vi "CRYReport Part ObjectClicked Event Callback.vi"(4 "TXTextControl":refnum<k7>, 5 "Event Data":cluster{"ObjectId":i16}, 6 "Control Ref":refnum<k7>, 7 "Event Common Data":T1) -> ()   [LabVIEW 2013]
uses:
  CRYReport Global.vi
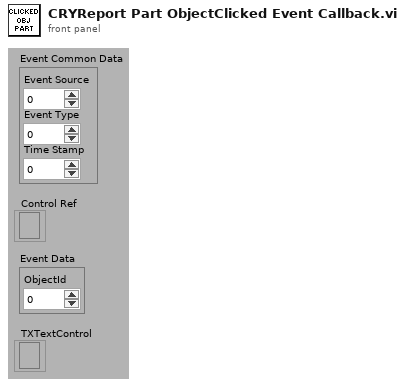
[diagram p1: front panel]
types:
  T1 = cluster{"Event Source":i32, "Event Type":u32, "Time Stamp":u32}
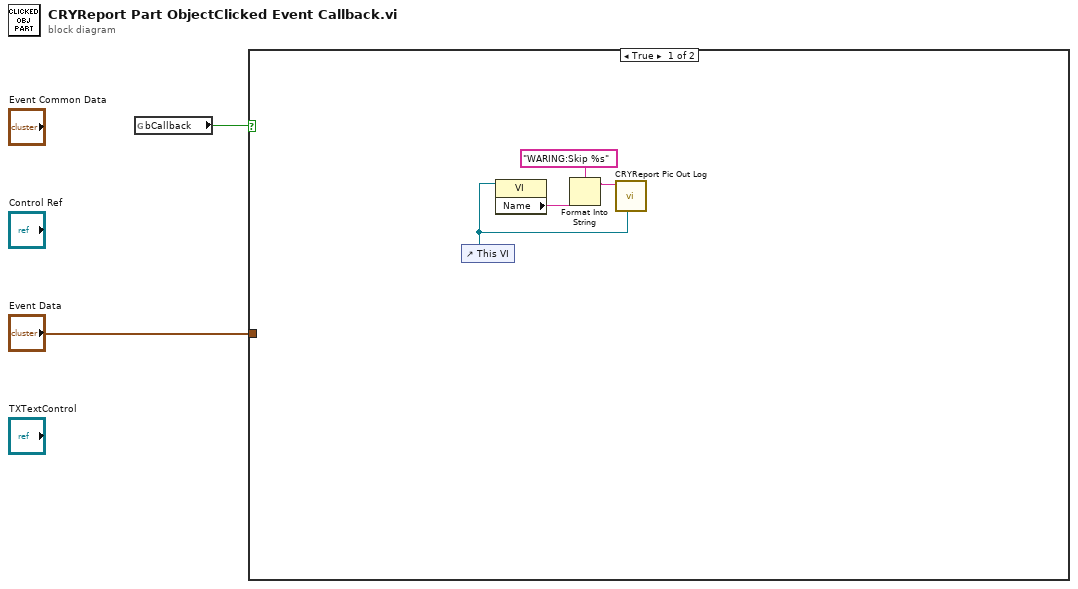
[diagram p0: block diagram]
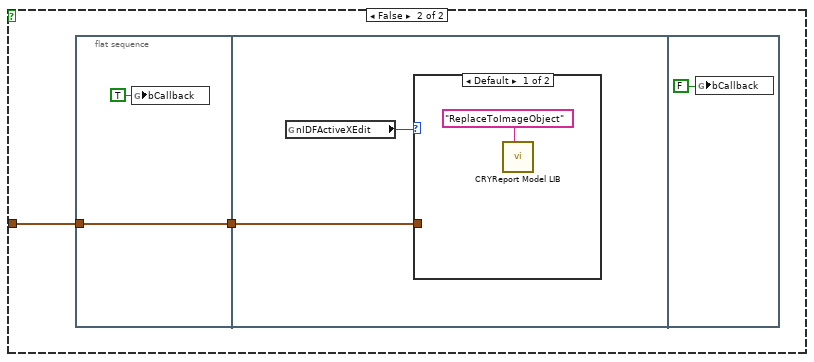
[diagram p2: hidden frame]
diagram:
  n1 = global read "CRYReport Global.vi" "bCallback"() -> (w1:bool)
  n2 = case shown="True" w1 {
    tunnel: "Event Data" -> [_ w7]
    frame True {
      n3 = control-ref of="This VI"() -> (w3:refnum<vi>)
      n4 = property class="VI"(reference=w3) -> ("Name"=w4:string)  [unwired: 1 in, 2 out]
      n5 = Format Into String(format string="WARING:Skip %s" ("string"), w4) -> (resulting string=w6:string)  [unwired: 2 in, 1 out]
      n6 = call "CRYReport Pic Out Log.vi"("vi reference"=w3, "sData"=w6) -> ()  [unwired: 10 in]
    }
    frame False {
      n7 = flat-sequence {
        tunnel: w7 -> [w10]
        tunnel: [w10] -> w8
        tunnel: w8 -> [w12]
        frame #0 {
          n8 = global write "CRYReport Global.vi" "bCallback"(TRUE ("bCallback")) -> ()
        }
        frame #1 {
          n9 = global read "CRYReport Global.vi" "nIDFActiveXEdit"() -> (w11:i16)
          n10 = case shown="Default" w11 {
            tunnel: w12 -> [_ _]
            frame Default {
              n11 = call "CRYReport Model LIB.vi"("sAction"="ReplaceToImageObject") -> ()  [unwired: 9 in, 2 out]
            }
            frame -1 {
            }
          }
        }
        frame #2 {
          n12 = global write "CRYReport Global.vi" "bCallback"(FALSE ("bCallback")) -> ()
        }
      }
    }
  }
